vi "Make Default settings.vi"() -> (3 "TD to be saved":T1={"Common properties"={"Measurement status ref"=refnum, "TWM Status ref"=refnum, "Abort ref"=refnum, "Skip waiting ref"=refnum, "GNU Octave path"=path "", "TWM+QWTB path"=path "", "lvlib path"=path "", "TWM pipe"="", "PJVS status ref"=refnum, "WAC path"=path ""}, "AC Source"={"AC Source type"=enum."Fluke 5XXX calibrator", "VISA"="", "Ref. clock (Hz)"=0.0, "status ref"=refnum, "Fluke 57XX wideband output"=FALSE, "Fluke 57XX ignore errors"=FALSE, "Synchronization by AC signal"=FALSE}, "DC meter"={"DC meter type"=enum."H/A/K 3458", "DC meter VISA"="", "NPLC"=0.0, "status ref"=refnum}, "CE measurement"={"Signal frequencies (Hz) T"=[], "Signal amplitudes (V) T"=[], "Sampling frequencies (Hz) T"=[], "Record lengths (multiples of periods) T"=[], "TWM data root directory"=path "", "TWM mreasurements directories"=[], "Calculate RMS from samples"=FALSE, "Algorithm to use"="", "Quantity to read"="TWM-WFFT", "Settle down after AC source change (s) T"=0.0, "Skip PJVS setup"=FALSE, "Measurement template file"=path "", "Row of START keyword T"=0, "Row of STOP keyword T"=0, "Measurement template line T"=[], "Switch position T"=[10000.0], "FR fit mat file T"=path "", "Recalculate-skip already calculated"=FALSE}, "FR measurement"={"Measurement frequencies (Hz)"=[], "Sampling frequency (Hz)"=0.0, "Signal amplitude (V)"=0.0, "AC-DC settle time (s)"=0.0, "Record length (multiples of period)"=[], "Measurement template file"=path "", "Row of START keyword"=0, "Row of STOP keyword"=0, "Calculate RMS from samples"=FALSE, "AC-DC warm up time (s)"=0.0, "Measurement template line"=[], "DC meter readings No."=0, "Algorithm"="", "Simultaneous measurement"=FALSE, "Recalculate-skip already calculated"=FALSE}, "FR template"={"Keywords column"=0, "Sig. freq. column"=0, "Rec. len. column"=0, "Meas. points. row min to read"=0, "Meas. points. row max to read"=0, "Properties column"=0, "Properties row start"=0, "Properties row end"=0, "Keyword START regexp"="", "Keyword STOP regexp"="", "HW data column"=0, "HW data row start"=0, "HW data row end"=0, "TIme and date column start"=0, "Digitizer value column start "=0, "DC mean column start "=0, "DC readings column start"=0}, "CE template"={"Keywords column"=0, "Sig. freq. column"=1, "Rec. len. column"=2, "Switch pos column"=3, "Meas. points. row min to read"=13, "Meas. points. row max to read"=1999, "Properties column"=4, "Properties row start"=1, "Properties row end"=7, "Keyword START regexp"="[Ss][Tt][Aa][Rr][Tt]", "Keyword STOP regexp"="[Ss][Tt][Oo][Pp]", "HW data column"=7, "HW data row start"=1, "HW data row end"=3, "TIme and date column start"=4, "Digitizer value column start "=5}, "PJVS"={"PJVS type"=enum."AC-supraVOLTcontrol", "Status Refnum"=refnum, "AC-supraVOLTcontrol"={"IP address:port (0.0.0.0:0000)"="0.0.0.0:0000", "Timeouts"={"TCP Read & Write (ms)"=7000, "Sensors readout"=5000, "PJVS setup"=10000, "Nullmeter readout"=5000, "Multiplexer setup"=3000, "57XX setup"=15000, "Generator setup"=5000, "Synthesizer setup"=3000, "Sampler readout"=10000}, "Simulation mode"=FALSE, "Debug mode"=FALSE}, "NPL bias source"={"DataSocketCluster"={"Server Machine"="CZC105BD8M", "Client Machine"="localhost", "Data"="P2", "TimeStamp"=0.0, "Count"=1, "Target Process"="General Server"}}, "Manual PJVS"={"PJVS frequency (Hz)"=0.0, "Reference voltages (V)"=[], "File with PJVS voltages"=path ""}, "VTT PJVS"={"some VTT only property"=""}}, "SS measurement"={"Signal frequencies (Hz)"=[1000.0], "Signal amplitudes (V)"=[0.707], "Sampling frequencies (Hz)"=[10000000.0], "Record lengths (multiples of periods)"=[10000.0], "Calculate results"=FALSE, "Algorithm"="TWM-WFFT", "TWM data directories"=[], "TWM data directories relative"=[], "Settle down after AC source change (s)"=1.0, "PJVS frequencies (Hz)"=[1000.0], "PJVS reference voltages array of vector cluster"=[{"PJVS reference voltages vector"=[]}], "Requested PJVS steps"=[20], "Measure CE"=FALSE, "Measure CE before"=FALSE, "Measure CE after"=FALSE, "Single point CE measurement"=FALSE, "original CE template path"=path "", "new CE template path before SS"=path "", "new CE template path before SS relative"=path "", "new CE template path after SS"=path "", "new CE template path after SS relative"=path "", "original CE fit path"=path "", "new CE fit path before SS"=path "", "new CE fit path before SS relative"=path "", "new CE fit path after SS"=path "", "new CE fit path after SS relative"=path "", "Measure digitizer gain"=FALSE, "Measure digitizer gain before"=FALSE, "Measure digitizer gain after"=FALSE, "Digitizer gain"=0.0, "Data folder"=path "", "FR fit path"=path "", "new FR fit path relative"=path "", "Rs"=0, "Re"=0, "SS measurement info files"=[]}, "AC sync source"={"AC Source type"=enum."Fluke 5XXX calibrator", "VISA"="", "Ref. clock (Hz)"=0.0, "status ref"=refnum, "Fluke 57XX wideband output"=FALSE, "Fluke 57XX ignore errors"=FALSE, "Synchronization by AC signal"=FALSE}, "DG measurement"={"Sampling frequencies (Hz)"=[10000000.0], "Requested PJVS frequencies (Hz)"=[1000.0], "Requested PJVS waveform amplitudes (V)"=[0.707], "Record lengths (multiples of PJVS periods)"=[10000.0], "Requested PJVS steps"=[20], "Switch position"=0.0, "Settle down after PJVS change (s)"=1.0, "Rs"=0, "Re"=0, "Algorithm"="TWM-PJVSSubS", "Calculate results"=FALSE, "Data folder"=path "", "TWM data directories"=[], "TWM data directories relative"=[], "DG measurement info files"=[], "Set PJVS frequencies (Hz)"=[1000.0], "Set PJVS reference voltages array of vector cluster"=[], "Set PJVS steps"=[1000]}} {"DG measurement"."Set PJVS frequencies (Hz)" format="%#_3p"; "DG measurement"."Set PJVS reference voltages array of vector cluster"."PJVS reference voltages vector" format="%#_3p"; "DG measurement"."Requested PJVS frequencies (Hz)" format="%#_3p"; "DG measurement"."Record lengths (multiples of PJVS periods)" format="%#_3p"; "DG measurement"."Sampling frequencies (Hz)" format="%#_3p"; "DG measurement"."Requested PJVS waveform amplitudes (V)" format="%#_3p"; "SS measurement"."PJVS reference voltages array of vector cluster"."PJVS reference voltages vector" format="%#_3p"; "SS measurement"."PJVS frequencies (Hz)" format="%#_3p"; "SS measurement"."Record lengths (multiples of periods)" format="%#_3p"; "SS measurement"."Sampling frequencies (Hz)" format="%#_3p"; "SS measurement"."Signal amplitudes (V)" format="%#_3p"; "SS measurement"."Signal frequencies (Hz)" format="%#_3p"; "PJVS"."NPL bias source"."DataSocketCluster"."TimeStamp" format="%.2f"; "CE measurement"."Switch position T" format="%#_3p"; "CE measurement"."Record lengths (multiples of periods) T" format="%#_3p"; "CE measurement"."Sampling frequencies (Hz) T" format="%#_3p"; "CE measurement"."Signal amplitudes (V) T" format="%#_3p"; "CE measurement"."Signal frequencies (Hz) T" format="%#_3p"; "FR measurement"."Record length (multiples of period)" format="%#_3p"; "FR measurement"."Sampling frequency (Hz)" format="%#_3p"; "FR measurement"."Measurement frequencies (Hz)" format="%#_3p"})   [LabVIEW 2020]
doc: "Returns QPS set to default values."
uses:
  Type definitions/Type definitions to be saved.ctl
  Type definitions/Common properties.ctl
  General AC source/Type definitions/AC Source.ctl
  General AC source/Type definitions/AC Source type.ctl
  General DC meter/Type definitions/DC meter.ctl
  General DC meter/Type definitions/DC meter type.ctl
  CE Measurement/Type definitions/CE measurement.ctl
  FR Measurement/Type definitions/FR measuement.ctl
  FR Utilities/Type definitions/FR template.ctl
  CE Utilities/Type definitions/CE template.ctl
  General PJVS driver/Type definitions/PJVS.ctl
  General PJVS driver/Type definitions/PJVS Type.ctl
  external libraries/acsvcontrol-driver/Public/Type Definitions/Timeouts.ctl
  external libraries/JV modified NPL Bias source/DataSocketCluster external.ctl
  SS Measurement/Type definitions/SS measurement.ctl
  DG Measurement/DG measurement.ctl
  <vilib>/Utility/sysdir.llb/System Directory Type.ctl
  external libraries/acsvcontrol-driver/ACSVcontrol-driver.lvlib
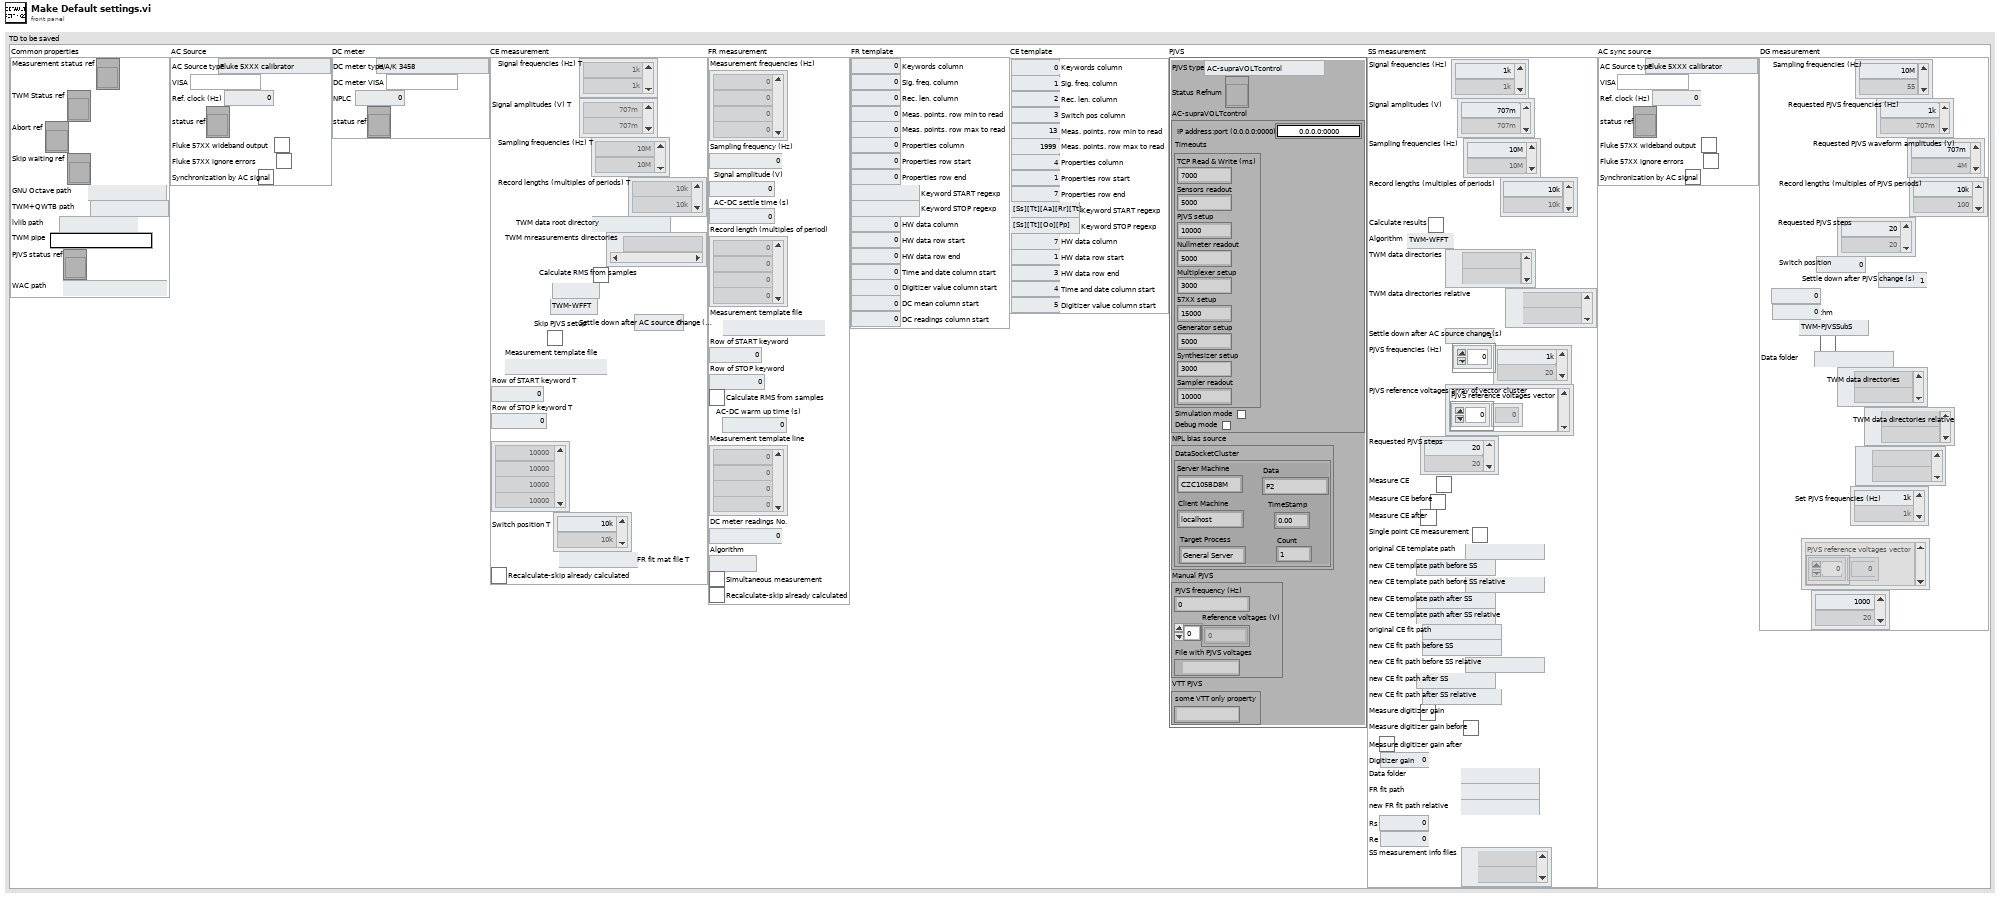
[diagram p1: front panel]
types:
  T1 = typedef "Type definitions to be saved.ctl" = cluster{"Common properties":T2, "AC Source":T3, "DC meter":T5, "CE measurement":T7, "FR measurement":T8, "FR template":T9, "CE template":T10, "PJVS":T11, "SS measurement":T15, "AC sync source":T3, "DG measurement":T16}
  T2 = typedef "Common properties.ctl" = cluster{"Measurement status ref":refnum<vi>, "TWM Status ref":refnum<vi>, "Abort ref":refnum<vi>, "Skip waiting ref":refnum<vi>, "GNU Octave path":path, "TWM+QWTB path":path, "lvlib path":path, "TWM pipe":string, "PJVS status ref":refnum<vi>, "WAC path":path}
  T3 = typedef "AC Source.ctl" = cluster{"AC Source type":T4, "VISA":refnum<visa-resource-name>, "Ref. clock (Hz)":dbl, "status ref":refnum<vi>, "Fluke 57XX wideband output":bool, "Fluke 57XX ignore errors":bool, "Synchronization by AC signal":bool}
  T4 = typedef "AC Source type.ctl" = enum16{"Fluke 5XXX calibrator", "Tektronix AFG3000 series", "dummy", "Agilent 331xxA to 332xxA", "Agilent 335xxA to 336xxA"}
  T5 = typedef "DC meter.ctl" = cluster{"DC meter type":T6, "DC meter VISA":refnum<visa-resource-name>, "NPLC":dbl, "status ref":refnum<vi>}
  T6 = typedef "DC meter type.ctl" = enum16{"H/A/K 3458", "Fluke 8508A", "dummy", "Keithley 2182"}
  T7 = typedef "CE measurement.ctl" = cluster{"Signal frequencies (Hz) T":dbl[], "Signal amplitudes (V) T":dbl[], "Sampling frequencies (Hz) T":dbl[], "Record lengths (multiples of periods) T":dbl[], "TWM data root directory":path, "TWM mreasurements directories":path[], "Calculate RMS from samples":bool, "Algorithm to use":string, "Quantity to read":string, "Settle down after AC source change (s) T":dbl, "Skip PJVS setup":bool, "Measurement template file":path, "Row of START keyword T":i32, "Row of STOP keyword T":i32, "Measurement template line T":i32[], "Switch position T":dbl[], "FR fit mat file T":path, "Recalculate-skip already calculated":bool}
  T8 = typedef "FR measuement.ctl" = cluster{"Measurement frequencies (Hz)":dbl[], "Sampling frequency (Hz)":dbl, "Signal amplitude (V)":dbl, "AC-DC settle time (s)":dbl, "Record length (multiples of period)":dbl[], "Measurement template file":path, "Row of START keyword":i32, "Row of STOP keyword":i32, "Calculate RMS from samples":bool, "AC-DC warm up time (s)":dbl, "Measurement template line":i32[], "DC meter readings No.":i32, "Algorithm":string, "Simultaneous measurement":bool, "Recalculate-skip already calculated":bool}
  T9 = typedef "FR template.ctl" = cluster{"Keywords column":i32, "Sig. freq. column":i32, "Rec. len. column":i32, "Meas. points. row min to read":i32, "Meas. points. row max to read":i32, "Properties column":i32, "Properties row start":i32, "Properties row end":i32, "Keyword START regexp":string, "Keyword STOP regexp":string, "HW data column":i32, "HW data row start":i32, "HW data row end":i32, "TIme and date column start":i32, "Digitizer value column start ":i32, "DC mean column start ":i32, "DC readings column start":i32}
  T10 = typedef "CE template.ctl" = cluster{"Keywords column":i32, "Sig. freq. column":i32, "Rec. len. column":i32, "Switch pos column":i32, "Meas. points. row min to read":i32, "Meas. points. row max to read":i32, "Properties column":i32, "Properties row start":i32, "Properties row end":i32, "Keyword START regexp":string, "Keyword STOP regexp":string, "HW data column":i32, "HW data row start":i32, "HW data row end":i32, "TIme and date column start":i32, "Digitizer value column start ":i32}
  T11 = typedef "PJVS.ctl" = cluster{"PJVS type":T12, "Status Refnum":refnum<vi>, "AC-supraVOLTcontrol":cluster{"IP address:port (0.0.0.0:0000)":string, "Timeouts":T13, "Simulation mode":bool, "Debug mode":bool}, "NPL bias source":cluster{"DataSocketCluster":T14}, "Manual PJVS":cluster{"PJVS frequency (Hz)":dbl, "Reference voltages (V)":dbl[], "File with PJVS voltages":path}, "VTT PJVS":cluster{"some VTT only property":string}}
  T12 = typedef "PJVS Type.ctl" = enum16{"AC-supraVOLTcontrol", "JV modified NPL bias control", "Manual PJVS", "VTT PJVS"}
  T13 = typedef "ACSVcontrol-driver.lvlib/Timeouts.ctl" = cluster{"TCP Read & Write (ms)":i32, "Sensors readout":i32, "PJVS setup":i32, "Nullmeter readout":i32, "Multiplexer setup":i32, "57XX setup":i32, "Generator setup":i32, "Synthesizer setup":i32, "Sampler readout":i32}
  T14 = typedef "DataSocketCluster external.ctl" = cluster{"Server Machine":string, "Client Machine":string, "Data":string, "TimeStamp":dbl, "Count":i32, "Target Process":string}
  T15 = typedef "SS measurement.ctl" = cluster{"Signal frequencies (Hz)":dbl[], "Signal amplitudes (V)":dbl[], "Sampling frequencies (Hz)":dbl[], "Record lengths (multiples of periods)":dbl[], "Calculate results":bool, "Algorithm":string, "TWM data directories":path[], "TWM data directories relative":path[], "Settle down after AC source change (s)":dbl, "PJVS frequencies (Hz)":dbl[], "PJVS reference voltages array of vector cluster":cluster{"PJVS reference voltages vector":dbl[]}[], "Requested PJVS steps":u32[], "Measure CE":bool, "Measure CE before":bool, "Measure CE after":bool, "Single point CE measurement":bool, "original CE template path":path, "new CE template path before SS":path, "new CE template path before SS relative":path, "new CE template path after SS":path, "new CE template path after SS relative":path, "original CE fit path":path, "new CE fit path before SS":path, "new CE fit path before SS relative":path, "new CE fit path after SS":path, "new CE fit path after SS relative":path, "Measure digitizer gain":bool, "Measure digitizer gain before":bool, "Measure digitizer gain after":bool, "Digitizer gain":dbl, "Data folder":path, "FR fit path":path, "new FR fit path relative":path, "Rs":i32, "Re":i32, "SS measurement info files":path[]}
  T16 = typedef "DG measurement.ctl" = cluster{"Sampling frequencies (Hz)":dbl[], "Requested PJVS frequencies (Hz)":dbl[], "Requested PJVS waveform amplitudes (V)":dbl[], "Record lengths (multiples of PJVS periods)":dbl[], "Requested PJVS steps":u32[], "Switch position":dbl, "Settle down after PJVS change (s)":dbl, "Rs":i32, "Re":i32, "Algorithm":string, "Calculate results":bool, "Data folder":path, "TWM data directories":path[], "TWM data directories relative":path[], "DG measurement info files":path[], "Set PJVS frequencies (Hz)":dbl[], "Set PJVS reference voltages array of vector cluster":cluster{"PJVS reference voltages vector":dbl[]}[], "Set PJVS steps":u32[]}
  T17 = cluster{"PJVS reference voltages vector":dbl[]}[]
  T18 = typedef "System Directory Type.ctl" = i32
  T19 = cluster{"PJVS frequency (Hz)":dbl, "Reference voltages (V)":dbl[], "File with PJVS voltages":path}
  T20 = cluster{"IP address:port (0.0.0.0:0000)":string, "Timeouts":T13, "Simulation mode":bool, "Debug mode":bool}
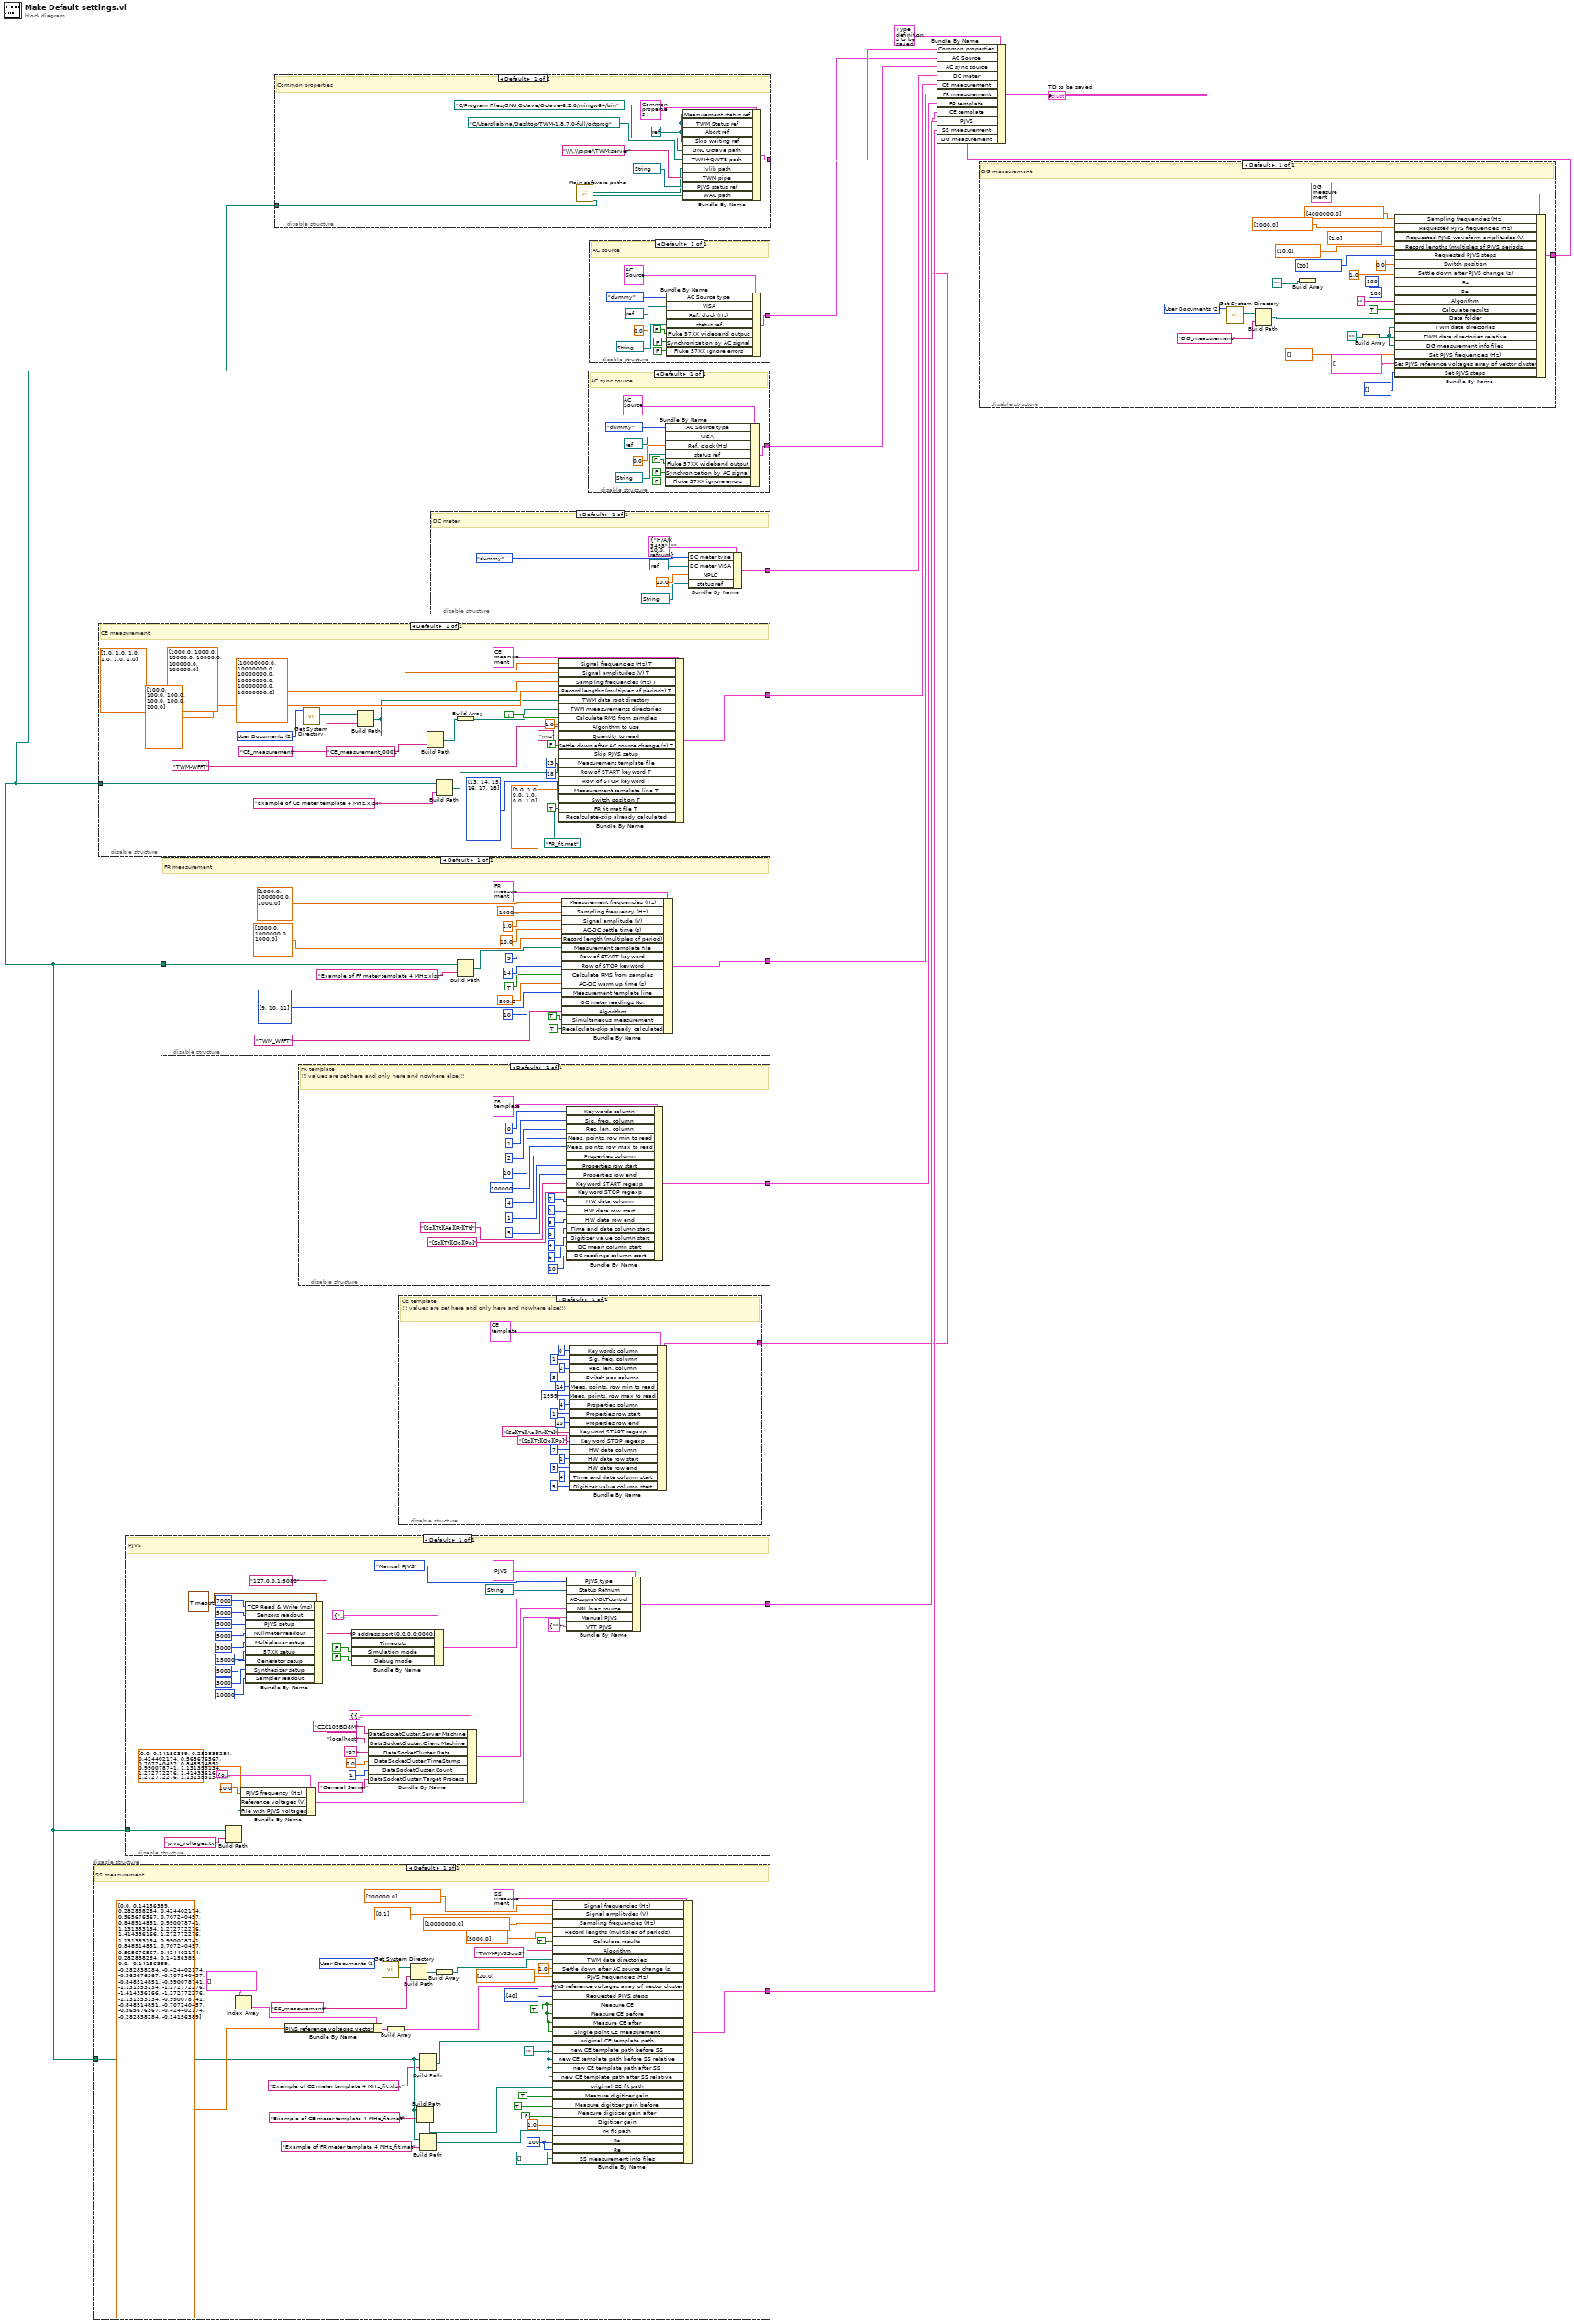
[diagram p0: block diagram]
diagram:
  n1 = disable-structure shown="Default" {
    disable-tunnel: [w19] -> w13
    disable-tunnel: [w15] -> w2
    frame Enabled {
      w23 = refnum<k0> refnum
      # "Common properties"
      n2 = call "Main software paths.vi"() -> ("templates dir path"=w15:path, "data processing dir path"=w17:path, "lv proc file path"=w16:path)  [unwired: 8 in, 1 out]
      n3 = Bundle By Name(cluster=T2 {"Measurement status ref"=refnum, "TWM Status ref"=refnum, "Abort ref"=refnum, "Skip waiting ref"=refnum, "GNU Octave path"=path "C:/Program Files/GNU Octave/Octave-6.2.0/mingw64/bin", "TWM+QWTB path"=path "C:/Users/labina/Desktop/TWM-1.8.7.0-full/octprog", "lvlib path"=path "D:/martin/WAC/WACsw - github/control_software/Filter function meter/external libraries/GOLPI 0.7.3.1 source distribution LV 20.0 32 bit/lv_proc.dll", "TWM pipe"="\\\\.\\pipe\\TWM:server", "PJVS status ref"=refnum, "WAC path"=path ""} ("Common properties"), "Measurement status ref"=w23, "TWM Status ref"=w23, "Abort ref"=w23, "Skip waiting ref"=w23, "GNU Octave path"=path "C:/Program Files/GNU Octave/Octave-6.2.0/mingw64/bin", "TWM+QWTB path"=path "C:/Users/labina/Desktop/TWM-1.8.7.0-full/octprog", "lvlib path"=w16, "TWM pipe"="\\\\.\\pipe\\TWM:server", "PJVS status ref"=refnum<vi> refnum, "WAC path"=w17) -> (w19:T2)
    }
  }
  n4 = disable-structure shown="Default" {
    disable-tunnel: [w47] -> w5
    disable-tunnel: w2 -> [w28]
    frame Enabled {
      (unwired) "Example of CE meter template 4 MHz_fit.mat" ("Algorithm")
      w29 = path ""
      w36 = 100 ("Rs")
      w45 = T18 2 items=["User Home"=0, "User Desktop"=1, "User Documents"=2, "User Application Data"=3, "User Preferences"=4, "User Temporary"=5, "Public Documents"=6, "Public Application Data"=7, "Public Preferences"=8, "Public Cache"=13, "System Core Libraries"=9, "System Installed Libraries"=10, "Application Files"=11, "Boot Volume Root"=12] ("system directory type")
      w30 = TRUE ("Measure CE")
      # "SS measurement"
      n5 = Index Array(array=T17 [] ("PJVS reference voltages array of vector cluster")) -> (element=w34:cluster{"PJVS reference voltages vector":dbl[]})  [unwired: 1 in]
      n6 = Bundle By Name(cluster=w34, "PJVS reference voltages vector"=dbl[] [0.0, 0.14156389, 0.282838284, 0.424402174, 0.565676567, 0.707240457, 0.848514851, 0.990078741, 1.131353134, 1.272772276, 1.414336166, 1.272772276, 1.131353134, 0.990078741, 0.848514851, 0.707240457, 0.565676567, 0.424402174, 0.282838284, 0.14156389, 0.0, -0.14156389, -0.282838284, -0.424402174, -0.565676567, -0.707240457, -0.848514851, -0.990078741, -1.131353134, -1.272772276, -1.414336166, -1.272772276, -1.131353134, -0.990078741, -0.848514851, -0.707240457, -0.565676567, -0.424402174, -0.282838284, -0.14156389] ("manual: reference voltages (V)")) -> (w32:cluster{"PJVS reference voltages vector":dbl[]})
      n7 = call <vilib>:"Get System Directory.vi"("system directory type"=w45) -> ("system directory"=w43:path)  [unwired: 10 in]
      n8 = Build Array(w32) -> (w31:T17)
      n9 = Build Path(base path=w43, name or relative path="SS_measurement" ("RMS algorithm")) -> (appended path=w42:path)
      n10 = Build Path(base path=w28, name or relative path="Example of CE meter template 4 MHz_fit.mat" ("Algorithm")) -> (appended path=w39:path)
      n11 = Build Path(base path=w28, name or relative path="Example of CE meter template 4 MHz_fit.xlsx" ("Algorithm")) -> (appended path=w26:path)
      n12 = Build Path(base path=w28, name or relative path="Example of FR meter template 4 MHz_fit.mat" ("Algorithm")) -> (appended path=w37:path)
      n13 = Build Array(w42) -> (w41:path[])
      n14 = Bundle By Name(cluster=T15 {"Signal frequencies (Hz)"=[1000.0], "Signal amplitudes (V)"=[0.707], "Sampling frequencies (Hz)"=[10000000.0], "Record lengths (multiples of periods)"=[10000.0], "Calculate results"=FALSE, "Algorithm"="TWM-WFFT", "TWM data directories"=[], "TWM data directories relative"=[], "Settle down after AC source change (s)"=1.0, "PJVS frequencies (Hz)"=[1000.0], "PJVS reference voltages array of vector cluster"=[{"PJVS reference voltages vector"=[]}], "Requested PJVS steps"=[20], "Measure CE"=FALSE, "Measure CE before"=FALSE, "Measure CE after"=FALSE, "Single point CE measurement"=FALSE, "original CE template path"=path "", "new CE template path before SS"=path "", "new CE template path before SS relative"=path "", "new CE template path after SS"=path "", "new CE template path after SS relative"=path "", "original CE fit path"=path "", "new CE fit path before SS"=path "", "new CE fit path before SS relative"=path "", "new CE fit path after SS"=path "", "new CE fit path after SS relative"=path "", "Measure digitizer gain"=FALSE, "Measure digitizer gain before"=FALSE, "Measure digitizer gain after"=FALSE, "Digitizer gain"=0.0, "Data folder"=path "", "FR fit path"=path "", "new FR fit path relative"=path "", "Rs"=0, "Re"=0, "SS measurement info files"=[]} ("SS measurement"), "Signal frequencies (Hz)"=dbl[] [100000.0], "Signal amplitudes (V)"=dbl[] [0.1], "Sampling frequencies (Hz)"=dbl[] [10000000.0], "Record lengths (multiples of periods)"=dbl[] [5000.0], "Calculate results"=TRUE, "Algorithm"="TWM-PJVSSubS", "TWM data directories"=w41, "Settle down after AC source change (s)"=1.0, "PJVS frequencies (Hz)"=dbl[] [20.0], "PJVS reference voltages array of vector cluster"=w31, "Requested PJVS steps"=u32[] [40], "Measure CE"=w30, "Measure CE before"=w30, "Measure CE after"=w30, "Single point CE measurement"=w30, "original CE template path"=w26, "new CE template path before SS"=w29, "new CE template path before SS relative"=w29, "new CE template path after SS"=w29, "new CE template path after SS relative"=w29, "original CE fit path"=w39, "Measure digitizer gain"=TRUE, "Measure digitizer gain before"=TRUE, "Measure digitizer gain after"=FALSE, "Digitizer gain"=1.0, "FR fit path"=w37, "Rs"=w36, "Re"=w36, "SS measurement info files"=path[] []) -> (w47:T15)
    }
  }
  n15 = disable-structure shown="Default" {
    disable-tunnel: [w79] -> w10
    disable-tunnel: w2 -> [w63]
    frame Enabled {
      w77 = T18 2 items=["User Home"=0, "User Desktop"=1, "User Documents"=2, "User Application Data"=3, "User Preferences"=4, "User Temporary"=5, "Public Documents"=6, "Public Application Data"=7, "Public Preferences"=8, "Public Cache"=13, "System Core Libraries"=9, "System Installed Libraries"=10, "Application Files"=11, "Boot Volume Root"=12] ("system directory type")
      # "CE measurement"
      n16 = call <vilib>:"Get System Directory.vi"("system directory type"=w77) -> ("system directory"=w76:path)  [unwired: 10 in]
      n17 = Build Path(base path=w76, name or relative path="CE_measurement" ("RMS algorithm")) -> (appended path=w72:path)
      n18 = Build Path(base path=w72, name or relative path="CE_measurement_0001" ("RMS algorithm")) -> (appended path=w73:path)
      n19 = Build Path(base path=w63, name or relative path="Example of CE meter template 4 MHz.xlsx" ("RMS algorithm")) -> (appended path=w70:path)
      n20 = Build Array(w73) -> (w75:path[])
      n21 = Bundle By Name(cluster=T7 {"Signal frequencies (Hz) T"=[1000.0], "Signal amplitudes (V) T"=[0.707], "Sampling frequencies (Hz) T"=[10000000.0], "Record lengths (multiples of periods) T"=[10000.0], "TWM data root directory"=path "", "TWM mreasurements directories"=[], "Calculate RMS from samples"=FALSE, "Algorithm to use"="TWM-WFFT", "Quantity to read"="TWM-WFFT", "Settle down after AC source change (s) T"=1.0, "Skip PJVS setup"=FALSE, "Measurement template file"=path "", "Row of START keyword T"=0, "Row of STOP keyword T"=0, "Measurement template line T"=[], "Switch position T"=[10000.0], "FR fit mat file T"=path "", "Recalculate-skip already calculated"=FALSE} ("CE measurement"), "Signal frequencies (Hz) T"=dbl[] [1000.0, 1000.0, 10000.0, 10000.0, 100000.0, 100000.0] ("Record lengths (multiples of periods)"), "Signal amplitudes (V) T"=dbl[] [1.0, 1.0, 1.0, 1.0, 1.0, 1.0] ("Record lengths (multiples of periods)"), "Sampling frequencies (Hz) T"=dbl[] [10000000.0, 10000000.0, 10000000.0, 10000000.0, 10000000.0, 10000000.0] ("Record lengths (multiples of periods)"), "Record lengths (multiples of periods) T"=dbl[] [100.0, 100.0, 100.0, 100.0, 100.0, 100.0] ("Record lengths (multiples of periods)"), "TWM data root directory"=w72, "TWM mreasurements directories"=w75, "Calculate RMS from samples"=TRUE, "Algorithm to use"="TWM-WFFT" ("RMS algorithm"), "Quantity to read"="rms", "Settle down after AC source change (s) T"=1.0 ("Settle down after AC source change (s)"), "Skip PJVS setup"=FALSE, "Measurement template file"=w70, "Row of START keyword T"=13 ("Row of START keyword"), "Row of STOP keyword T"=18 ("Row of STOP keyword"), "Measurement template line T"=i32[] [13, 14, 15, 16, 17, 18] ("Measurement template line"), "Switch position T"=dbl[] [0.0, 1.0, 0.0, 1.0, 0.0, 1.0] ("Switch position"), "FR fit mat file T"=path "FR_fit.mat" ("FR fit mat file"), "Recalculate-skip already calculated"=TRUE) -> (w79:T7)
    }
  }
  n22 = disable-structure shown="Default" {
    disable-tunnel: [w98] -> w6
    disable-tunnel: w2 -> [w90]
    frame Enabled {
      # "PJVS"
      n23 = Build Path(base path=w90, name or relative path="pjvs_voltages.txt" ("DataSocketCluster.Server Machine")) -> (appended path=w89:path)
      n24 = Bundle By Name(cluster=T19 {"PJVS frequency (Hz)"=0.0, "Reference voltages (V)"=[], "File with PJVS voltages"=path ""} ("Manual PJVS"), "PJVS frequency (Hz)"=20.0, "Reference voltages (V)"=dbl[] [0.0, 0.14156389, 0.282838284, 0.424402174, 0.565676567, 0.707240457, 0.848514851, 0.990078741, 1.131353134, 1.272772276, 1.414336166, 1.272772276, 1.131353134, 0.990078741, 0.848514851, 0.707240457, 0.565676567, 0.424402174, 0.282838284, 0.14156389, 0.0, -0.14156389, -0.282838284, -0.424402174, -0.565676567, -0.707240457, -0.848514851, -0.990078741, -1.131353134, -1.272772276, -1.414336166, -1.272772276, -1.131353134, -0.990078741, -0.848514851, -0.707240457, -0.565676567, -0.424402174, -0.282838284, -0.14156389] ("manual: reference voltages (V)"), "File with PJVS voltages"=w89) -> (w101:T19)
      n25 = Bundle By Name(cluster=T13 {"TCP Read & Write (ms)"=7000, "Sensors readout"=5000, "PJVS setup"=5000, "Nullmeter readout"=5000, "Multiplexer setup"=3000, "57XX setup"=15000, "Generator setup"=5000, "Synthesizer setup"=3000, "Sampler readout"=10000} ("Timeouts"), "TCP Read & Write (ms)"=7000, "Sensors readout"=5000, "PJVS setup"=5000, "Nullmeter readout"=5000, "Multiplexer setup"=3000, "57XX setup"=15000, "Generator setup"=5000, "Synthesizer setup"=3000, "Sampler readout"=10000) -> (w114:T13)
      n26 = Bundle By Name(cluster=T20 {"IP address:port (0.0.0.0:0000)"="", "Timeouts"={"TCP Read & Write (ms)"=0, "Sensors readout"=0, "PJVS setup"=0, "Nullmeter readout"=0, "Multiplexer setup"=0, "57XX setup"=0, "Generator setup"=0, "Synthesizer setup"=0, "Sampler readout"=0}, "Simulation mode"=FALSE, "Debug mode"=FALSE} ("AC-supraVOLTcontrol"), "IP address:port (0.0.0.0:0000)"="127.0.0.1:8080", "Timeouts"=w114, "Simulation mode"=FALSE, "Debug mode"=FALSE) -> (w119:T20)
      n27 = Bundle By Name(cluster=cluster{"DataSocketCluster":T14} {"DataSocketCluster"={"Server Machine"="", "Client Machine"="", "Data"="", "TimeStamp"=0.0, "Count"=0, "Target Process"=""}} ("NPL bias source"), "DataSocketCluster.Server Machine"="CZC105BD8M", "DataSocketCluster.Client Machine"="localhost", "DataSocketCluster.Data"="P2", "DataSocketCluster.TimeStamp"=0.0, "DataSocketCluster.Count"=1, "DataSocketCluster.Target Process"="General Server") -> (w103:cluster{"DataSocketCluster":T14})
      n28 = Bundle By Name(cluster=T11 {"PJVS type"=enum."AC-supraVOLTcontrol", "Status Refnum"=refnum, "AC-supraVOLTcontrol"={"IP address:port (0.0.0.0:0000)"="0.0.0.0:0000", "Timeouts"={"TCP Read & Write (ms)"=7000, "Sensors readout"=5000, "PJVS setup"=10000, "Nullmeter readout"=5000, "Multiplexer setup"=3000, "57XX setup"=15000, "Generator setup"=5000, "Synthesizer setup"=3000, "Sampler readout"=10000}, "Simulation mode"=FALSE, "Debug mode"=FALSE}, "NPL bias source"={"DataSocketCluster"={"Server Machine"="CZC105BD8M", "Client Machine"="localhost", "Data"="P2", "TimeStamp"=0.0, "Count"=1, "Target Process"="General Server"}}, "Manual PJVS"={"PJVS frequency (Hz)"=0.0, "Reference voltages (V)"=[], "File with PJVS voltages"=path ""}, "VTT PJVS"={"some VTT only property"=""}} ("PJVS"), "PJVS type"=PJVS_Type."Manual PJVS", "Status Refnum"=refnum<vi> refnum ("status ref"), "AC-supraVOLTcontrol"=w119, "NPL bias source"=w103, "Manual PJVS"=w101, "VTT PJVS"=cluster{"some VTT only property":string} {"some VTT only property"=""}) -> (w98:T11)
    }
  }
  n29 = disable-structure shown="Default" {
    disable-tunnel: [w127] -> w9
    disable-tunnel: w2 -> [w124]
    frame Enabled {
      # "FR measurement"
      n30 = Build Path(base path=w124, name or relative path="Example of FF meter template 4 MHz.xlsx" ("Algorithm")) -> (appended path=w135:path)
      n31 = Bundle By Name(cluster=T8 {"Measurement frequencies (Hz)"=[1000.0, 10000.0, 1000.0], "Sampling frequency (Hz)"=500000.0, "Signal amplitude (V)"=4.5, "AC-DC settle time (s)"=20.0, "Record length (multiples of period)"=[1000.0, 10000.0, 1000.0], "Measurement template file"=path "", "Row of START keyword"=0, "Row of STOP keyword"=0, "Calculate RMS from samples"=FALSE, "AC-DC warm up time (s)"=300.0, "Measurement template line"=[], "DC meter readings No."=10, "Algorithm"="TWM-WFFT", "Simultaneous measurement"=FALSE, "Recalculate-skip already calculated"=FALSE} ("FR measurement"), "Measurement frequencies (Hz)"=dbl[] [1000.0, 1000000.0, 1000.0], "Sampling frequency (Hz)"=10000000.0, "Signal amplitude (V)"=1.0, "AC-DC settle time (s)"=10.0, "Record length (multiples of period)"=dbl[] [1000.0, 1000000.0, 1000.0], "Measurement template file"=w135, "Row of START keyword"=9, "Row of STOP keyword"=14, "Calculate RMS from samples"=TRUE, "AC-DC warm up time (s)"=300.0, "Measurement template line"=i32[] [9, 10, 11], "DC meter readings No."=10 ("No of readings"), "Algorithm"="TWM_WFFT", "Simultaneous measurement"=TRUE, "Recalculate-skip already calculated"=TRUE) -> (w127:T8)
    }
  }
  n32 = disable-structure shown="Default" {
    disable-tunnel: [w143] -> w8
    frame Enabled {
      # "FR template\n!!! values are set here and only here and nowhere else!!!"
      n33 = Bundle By Name(cluster=T9 {"Keywords column"=0, "Sig. freq. column"=1, "Rec. len. column"=2, "Meas. points. row min to read"=13, "Meas. points. row max to read"=1999, "Properties column"=4, "Properties row start"=1, "Properties row end"=7, "Keyword START regexp"="[Ss][Tt][Aa][Rr][Tt]", "Keyword STOP regexp"="[Ss][Tt][Oo][Pp]", "HW data column"=7, "HW data row start"=1, "HW data row end"=3, "TIme and date column start"=3, "Digitizer value column start "=4, "DC mean column start "=6, "DC readings column start"=10} ("FR template"), "Keywords column"=0, "Sig. freq. column"=1, "Rec. len. column"=2, "Meas. points. row min to read"=10, "Meas. points. row max to read"=100000, "Properties column"=4, "Properties row start"=1, "Properties row end"=5, "Keyword START regexp"="[Ss][Tt][Aa][Rr][Tt]", "Keyword STOP regexp"="[Ss][Tt][Oo][Pp]", "HW data column"=7, "HW data row start"=1, "HW data row end"=3, "TIme and date column start"=3, "Digitizer value column start"=4, "DC mean column start"=6, "DC readings column start"=10) -> (w143:T9)
    }
  }
  n34 = disable-structure shown="Default" {
    disable-tunnel: [w162] -> w4
    frame Enabled {
      # "CE template\n!!! values are set here and only here and nowhere else!!!"
      n35 = Bundle By Name(cluster=T10 {"Keywords column"=0, "Sig. freq. column"=1, "Rec. len. column"=2, "Switch pos column"=3, "Meas. points. row min to read"=13, "Meas. points. row max to read"=1999, "Properties column"=4, "Properties row start"=1, "Properties row end"=7, "Keyword START regexp"="[Ss][Tt][Aa][Rr][Tt]", "Keyword STOP regexp"="[Ss][Tt][Oo][Pp]", "HW data column"=7, "HW data row start"=1, "HW data row end"=3, "TIme and date column start"=4, "Digitizer value column start "=5} ("CE template"), "Keywords column"=0, "Sig. freq. column"=1, "Rec. len. column"=2, "Switch pos column"=3, "Meas. points. row min to read"=14, "Meas. points. row max to read"=1999, "Properties column"=4, "Properties row start"=1, "Properties row end"=10, "Keyword START regexp"="[Ss][Tt][Aa][Rr][Tt]", "Keyword STOP regexp"="[Ss][Tt][Oo][Pp]", "HW data column"=7, "HW data row start"=1, "HW data row end"=3, "TIme and date column start"=4, "Digitizer value column start"=5) -> (w162:T10)
    }
  }
  n36 = disable-structure shown="Default" {
    disable-tunnel: [w180] -> w11
    frame Enabled {
      # "DC meter"
      n37 = Bundle By Name(cluster=T5 {"DC meter type"=enum."H/A/K 3458", "DC meter VISA"="", "NPLC"=10.0, "status ref"=refnum} ("DC meter"), "DC meter type"=DC_meter_type."dummy", "DC meter VISA"=refnum<visa-resource-name> refnum, "NPLC"=10.0, "status ref"=refnum<vi> refnum) -> (w180:T5)
    }
  }
  n38 = disable-structure shown="Default" {
    disable-tunnel: [w189] -> w3
    frame Enabled {
      # "AC sync source"
      n39 = Bundle By Name(cluster=T3 {"AC Source type"=enum."Fluke 5XXX calibrator", "VISA"="", "Ref. clock (Hz)"=0.0, "status ref"=refnum, "Fluke 57XX wideband output"=FALSE, "Fluke 57XX ignore errors"=FALSE, "Synchronization by AC signal"=FALSE} ("AC Source"), "AC Source type"=AC_Source_type."dummy" ("AWG type"), "VISA"=refnum<visa-resource-name> refnum, "Ref. clock (Hz)"=0.0, "status ref"=refnum<vi> refnum, "Fluke 57XX wideband output"=FALSE, "Synchronization by AC signal"=FALSE, "Fluke 57XX ignore errors"=FALSE) -> (w189:T3)
    }
  }
  n40 = disable-structure shown="Default" {
    disable-tunnel: [w198] -> w12
    frame Enabled {
      # "AC source"
      n41 = Bundle By Name(cluster=T3 {"AC Source type"=enum."Fluke 5XXX calibrator", "VISA"="", "Ref. clock (Hz)"=0.0, "status ref"=refnum, "Fluke 57XX wideband output"=FALSE, "Fluke 57XX ignore errors"=FALSE, "Synchronization by AC signal"=FALSE} ("AC Source"), "AC Source type"=AC_Source_type."dummy" ("AWG type"), "VISA"=refnum<visa-resource-name> refnum, "Ref. clock (Hz)"=0.0, "status ref"=refnum<vi> refnum, "Fluke 57XX wideband output"=FALSE, "Synchronization by AC signal"=FALSE, "Fluke 57XX ignore errors"=FALSE) -> (w198:T3)
    }
  }
  n42 = disable-structure shown="Default" {
    disable-tunnel: [w225] -> w1
    frame Enabled {
      w222 = T18 2 items=["User Home"=0, "User Desktop"=1, "User Documents"=2, "User Application Data"=3, "User Preferences"=4, "User Temporary"=5, "Public Documents"=6, "Public Application Data"=7, "Public Preferences"=8, "Public Cache"=13, "System Core Libraries"=9, "System Installed Libraries"=10, "Application Files"=11, "Boot Volume Root"=12] ("system directory type")
      # "DG measurement"
      n43 = call <vilib>:"Get System Directory.vi"("system directory type"=w222) -> ("system directory"=w224:path)  [unwired: 10 in]
      n44 = Build Path(base path=w224, name or relative path="DG_measurement" ("RMS algorithm")) -> (appended path=w204:path)
      n45 = Build Array(path "") -> ()  [unwired: 1 out]
      n46 = Build Array(path "") -> (w215:path[])
      n47 = Bundle By Name(cluster=T16 {"Sampling frequencies (Hz)"=[10000000.0], "Requested PJVS frequencies (Hz)"=[1000.0], "Requested PJVS waveform amplitudes (V)"=[0.707], "Record lengths (multiples of PJVS periods)"=[10000.0], "Requested PJVS steps"=[20], "Switch position"=0.0, "Settle down after PJVS change (s)"=1.0, "Rs"=0, "Re"=0, "Algorithm"="TWM-PJVSSubS", "Calculate results"=FALSE, "Data folder"=path "", "TWM data directories"=[], "TWM data directories relative"=[], "DG measurement info files"=[], "Set PJVS frequencies (Hz)"=[1000.0], "Set PJVS reference voltages array of vector cluster"=[], "Set PJVS steps"=[1000]} ("DG measurement"), "Sampling frequencies (Hz)"=dbl[] [4000000.0], "Requested PJVS frequencies (Hz)"=dbl[] [1000.0] ("Signal frequencies (Hz)"), "Requested PJVS waveform amplitudes (V)"=dbl[] [1.0] ("PJVS amplitudes (Hz)"), "Record lengths (multiples of PJVS periods)"=dbl[] [10.0] ("Record lengths (multiples of periods)"), "Requested PJVS steps"=u32[] [20], "Switch position"=0.0, "Settle down after PJVS change (s)"=1.0, "Rs"=100, "Re"=100, "Algorithm"="", "Calculate results"=TRUE, "Data folder"=w204, "TWM data directories"=w215, "TWM data directories relative"=w215, "DG measurement info files"=w215, "Set PJVS frequencies (Hz)"=dbl[] [], "Set PJVS reference voltages array of vector cluster"=T17 [] ("PJVS reference voltages array of vector cluster"), "Set PJVS steps"=u32[] []) -> (w225:T16)
    }
  }
  n48 = Bundle By Name(cluster=T1 {"Common properties"={"Measurement status ref"=refnum, "TWM Status ref"=refnum, "Abort ref"=refnum, "Skip waiting ref"=refnum, "GNU Octave path"=path "", "TWM+QWTB path"=path "", "lvlib path"=path "", "TWM pipe"="", "PJVS status ref"=refnum, "WAC path"=path ""}, "AC Source"={"AC Source type"=enum."Fluke 5XXX calibrator", "VISA"="", "Ref. clock (Hz)"=0.0, "status ref"=refnum, "Fluke 57XX wideband output"=FALSE, "Fluke 57XX ignore errors"=FALSE, "Synchronization by AC signal"=FALSE}, "DC meter"={"DC meter type"=enum."H/A/K 3458", "DC meter VISA"="", "NPLC"=0.0, "status ref"=refnum}, "CE measurement"={"Signal frequencies (Hz) T"=[], "Signal amplitudes (V) T"=[], "Sampling frequencies (Hz) T"=[], "Record lengths (multiples of periods) T"=[], "TWM data root directory"=path "", "TWM mreasurements directories"=[], "Calculate RMS from samples"=FALSE, "Algorithm to use"="", "Quantity to read"="TWM-WFFT", "Settle down after AC source change (s) T"=0.0, "Skip PJVS setup"=FALSE, "Measurement template file"=path "", "Row of START keyword T"=0, "Row of STOP keyword T"=0, "Measurement template line T"=[], "Switch position T"=[10000.0], "FR fit mat file T"=path "", "Recalculate-skip already calculated"=FALSE}, "FR measurement"={"Measurement frequencies (Hz)"=[], "Sampling frequency (Hz)"=0.0, "Signal amplitude (V)"=0.0, "AC-DC settle time (s)"=0.0, "Record length (multiples of period)"=[], "Measurement template file"=path "", "Row of START keyword"=0, "Row of STOP keyword"=0, "Calculate RMS from samples"=FALSE, "AC-DC warm up time (s)"=0.0, "Measurement template line"=[], "DC meter readings No."=0, "Algorithm"="", "Simultaneous measurement"=FALSE, "Recalculate-skip already calculated"=FALSE}, "FR template"={"Keywords column"=0, "Sig. freq. column"=0, "Rec. len. column"=0, "Meas. points. row min to read"=0, "Meas. points. row max to read"=0, "Properties column"=0, "Properties row start"=0, "Properties row end"=0, "Keyword START regexp"="", "Keyword STOP regexp"="", "HW data column"=0, "HW data row start"=0, "HW data row end"=0, "TIme and date column start"=0, "Digitizer value column start "=0, "DC mean column start "=0, "DC readings column start"=0}, "CE template"={"Keywords column"=0, "Sig. freq. column"=1, "Rec. len. column"=2, "Switch pos column"=3, "Meas. points. row min to read"=13, "Meas. points. row max to read"=1999, "Properties column"=4, "Properties row start"=1, "Properties row end"=7, "Keyword START regexp"="[Ss][Tt][Aa][Rr][Tt]", "Keyword STOP regexp"="[Ss][Tt][Oo][Pp]", "HW data column"=7, "HW data row start"=1, "HW data row end"=3, "TIme and date column start"=4, "Digitizer value column start "=5}, "PJVS"={"PJVS type"=enum."AC-supraVOLTcontrol", "Status Refnum"=refnum, "AC-supraVOLTcontrol"={"IP address:port (0.0.0.0:0000)"="0.0.0.0:0000", "Timeouts"={"TCP Read & Write (ms)"=7000, "Sensors readout"=5000, "PJVS setup"=10000, "Nullmeter readout"=5000, "Multiplexer setup"=3000, "57XX setup"=15000, "Generator setup"=5000, "Synthesizer setup"=3000, "Sampler readout"=10000}, "Simulation mode"=FALSE, "Debug mode"=FALSE}, "NPL bias source"={"DataSocketCluster"={"Server Machine"="CZC105BD8M", "Client Machine"="localhost", "Data"="P2", "TimeStamp"=0.0, "Count"=1, "Target Process"="General Server"}}, "Manual PJVS"={"PJVS frequency (Hz)"=0.0, "Reference voltages (V)"=[], "File with PJVS voltages"=path ""}, "VTT PJVS"={"some VTT only property"=""}}, "SS measurement"={"Signal frequencies (Hz)"=[1000.0], "Signal amplitudes (V)"=[0.707], "Sampling frequencies (Hz)"=[10000000.0], "Record lengths (multiples of periods)"=[10000.0], "Calculate results"=FALSE, "Algorithm"="TWM-WFFT", "TWM data directories"=[], "TWM data directories relative"=[], "Settle down after AC source change (s)"=1.0, "PJVS frequencies (Hz)"=[1000.0], "PJVS reference voltages array of vector cluster"=[{"PJVS reference voltages vector"=[]}], "Requested PJVS steps"=[20], "Measure CE"=FALSE, "Measure CE before"=FALSE, "Measure CE after"=FALSE, "Single point CE measurement"=FALSE, "original CE template path"=path "", "new CE template path before SS"=path "", "new CE template path before SS relative"=path "", "new CE template path after SS"=path "", "new CE template path after SS relative"=path "", "original CE fit path"=path "", "new CE fit path before SS"=path "", "new CE fit path before SS relative"=path "", "new CE fit path after SS"=path "", "new CE fit path after SS relative"=path "", "Measure digitizer gain"=FALSE, "Measure digitizer gain before"=FALSE, "Measure digitizer gain after"=FALSE, "Digitizer gain"=0.0, "Data folder"=path "", "FR fit path"=path "", "new FR fit path relative"=path "", "Rs"=0, "Re"=0, "SS measurement info files"=[]}, "AC sync source"={"AC Source type"=enum."Fluke 5XXX calibrator", "VISA"="", "Ref. clock (Hz)"=0.0, "status ref"=refnum, "Fluke 57XX wideband output"=FALSE, "Fluke 57XX ignore errors"=FALSE, "Synchronization by AC signal"=FALSE}, "DG measurement"={"Sampling frequencies (Hz)"=[10000000.0], "Requested PJVS frequencies (Hz)"=[1000.0], "Requested PJVS waveform amplitudes (V)"=[0.707], "Record lengths (multiples of PJVS periods)"=[10000.0], "Requested PJVS steps"=[20], "Switch position"=0.0, "Settle down after PJVS change (s)"=1.0, "Rs"=0, "Re"=0, "Algorithm"="TWM-PJVSSubS", "Calculate results"=FALSE, "Data folder"=path "", "TWM data directories"=[], "TWM data directories relative"=[], "DG measurement info files"=[], "Set PJVS frequencies (Hz)"=[1000.0], "Set PJVS reference voltages array of vector cluster"=[], "Set PJVS steps"=[1000]}} ("TD to be saved"), "Common properties"=w13, "AC Source"=w12, "AC sync source"=w3, "DC meter"=w11, "CE measurement"=w10, "FR measurement"=w9, "FR template"=w8, "CE template"=w4, "PJVS"=w6, "SS measurement"=w5, "DG measurement"=w1) -> (→"TD to be saved":T1)
